vi "Save Image Data to File.vi"(5 "Image Format":enum16{"JPEG", "PNG", "BMP"}(ring), 8 "error in (no error)":errorcluster, 10 "image data":T1, 11 "Path":path) -> (0 "error out":errorcluster, 3 "Path Out":path)   [LabVIEW 2011]
uses:
  <vilib>/picture/picture.llb/imagedata.ctl
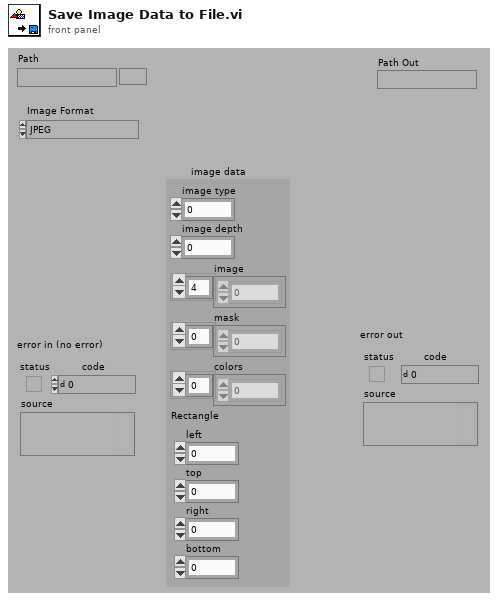
[diagram p1: front panel]
types:
  T1 = typedef "imagedata.ctl" = cluster{"image type":i32, "image depth":i32, "image":u8[], "mask":u8[], "colors":u32[], "Rectangle":cluster{"left":i16, "top":i16, "right":i16, "bottom":i16}}
  T2 = enum32{"existing file", "new file", "new or existing file", "existing dir", "new dir", "new or existing dir", "existing file (use LLBs)", "new file (use LLBs)", "new or existing file (use LLBs)", "new or existing file or directory (use LLBs)"}
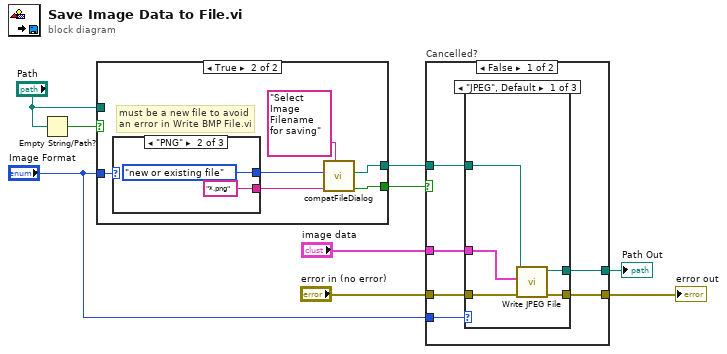
[diagram p0: block diagram]
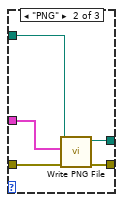
[diagram p2: hidden frame]
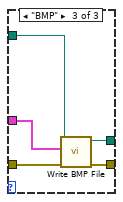
[diagram p3: hidden frame]
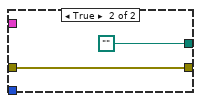
[diagram p4: hidden frame]
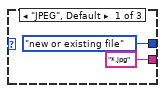
[diagram p6: hidden frame]
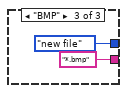
[diagram p7: hidden frame]
diagram:
  n1 = Empty String/Path?(string/path="Path") -> (empty?=w6:bool)
  n2 = case shown="True" w6 {
    selector: w6 -> [w10 _]
    tunnel: "Image Format" -> [_ w16]
    tunnel: [w11 w13] -> w2
    tunnel: "Path" -> [w11 _]
    tunnel: [w10 w12] -> w3
    frame False {
    }
    frame True {
      # "must be a new file to avoid\nan error in Write BMP File.vi"
      n3 = case shown="\"PNG\"" w16 {
        tunnel: ["*.jpg" ("pattern") "*.png" ("pattern") "*.bmp" ("pattern")] -> w14
        tunnel: [T2."new or existing file" ("select mode (2)") T2."new or existing file" ("select mode (2)") T2."new file" ("select mode (2)")] -> w15
        frame "JPEG", Default {
        }
        frame "PNG" {
        }
        frame "BMP" {
        }
      }
      n4 = call <vilib>:"compatFileDialog.vi"("prompt"="Select Image Filename for saving", "pattern"=w14, "select mode (2)"=w15) -> ("cancelled"=w12:bool, "path"=w13:path)  [unwired: 4 in, 3 out]
    }
  }
  n5 = case "Cancelled?" shown="False" w3 {
    tunnel: [w29 path ""] -> w9
    tunnel: "error in (no error)" -> [w28 w45]
    tunnel: [w27 w45] -> w7
    tunnel: "Image Format" -> [w26 _]
    tunnel: w2 -> [w25 _]
    tunnel: "image data" -> [w24 _]
    frame False {
      n6 = case shown="\"JPEG\", Default" w26 {
        tunnel: [w31 w38 w43] -> w29
        tunnel: w28 -> [w33 w36 w41]
        tunnel: [w32 w37 w42] -> w27
        tunnel: w25 -> [w34 w39 w44]
        tunnel: w24 -> [w30 w35 w40]
        frame "JPEG", Default {
          n7 = call <vilib>:"Write JPEG File.vi"("error in (no error)"=w33, "image data"=w30, "path to JPEG file"=w34) -> ("error out"=w32:errorcluster, "path"=w31:path)  [unwired: 7 out]
        }
        frame "PNG" {
          n8 = call <vilib>:"Write PNG File.vi"("error in (no error)"=w36, "image data"=w35, "path to PNG file"=w39) -> ("error out"=w37:errorcluster, "path"=w38:path)  [unwired: 7 out]
        }
        frame "BMP" {
          n9 = call <vilib>:"Write BMP File.vi"("error in (no error)"=w41, "image data"=w40, "path to BMP file"=w44) -> ("error out"=w42:errorcluster, "path"=w43:path)  [unwired: 7 out]
        }
      }
    }
    frame True {
    }
  }
  "Path Out" <- w9
  "error out" <- w7
